vi "Build Create Parameters.vi"(4 "TypeMap in":refnum<class "TypeMap.lvclass">, 8 "error in (no error)":errorcluster, 10 "object":variant, 11 "SqlMapper in":refnum<class "SqlMapper.lvclass">) -> (0 "error out":errorcluster, 1 "DynamicParameters out":refnum<class "DynamicParameters.lvclass">, 3 "SqlMapper out":refnum<class "SqlMapper.lvclass">)   [LabVIEW 2020, in "ORM.lvlib" / "TypeMap.lvclass"]
uses:
  TypeMap.lvclass
  DynamicParameters/DynamicParameters.lvclass
  SqlMapper/SqlMapper.lvclass
  TypeMap.lvclass/TypeMap.ctl
  Read Autokey.vi
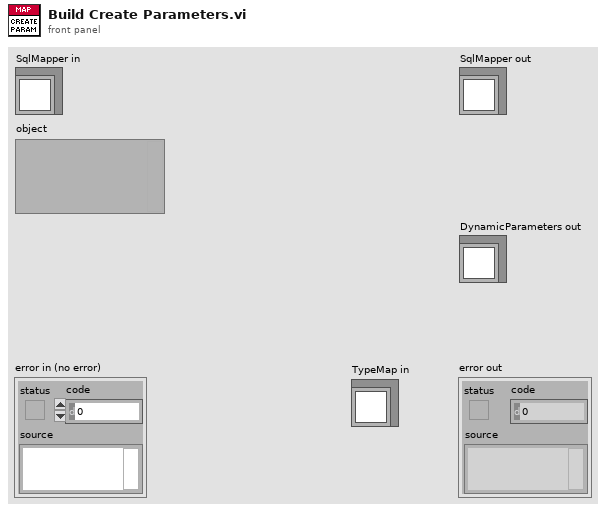
[diagram p1: front panel]
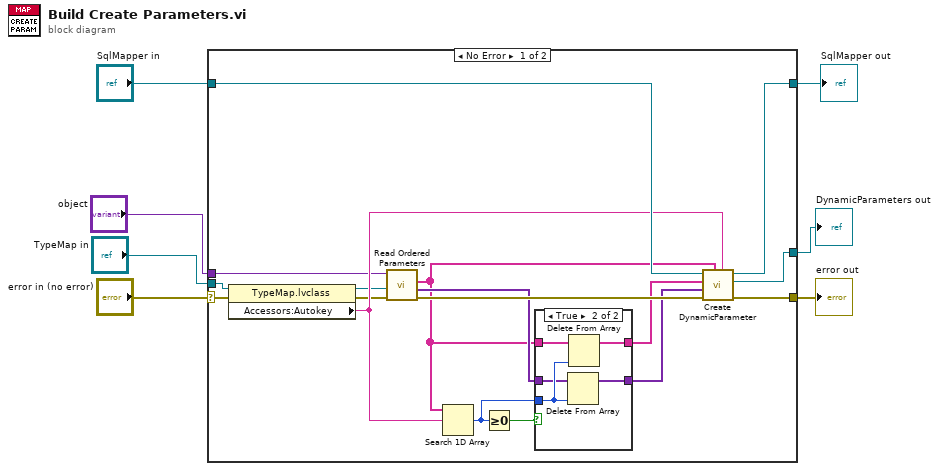
[diagram p0: block diagram]
diagram:
  n1 = case shown="No Error" "error in (no error)" {
    selector: "error in (no error)" -> [w22 w33]
    tunnel: [w14 w33] -> w6
    tunnel: "TypeMap in" -> [w24 _]
    tunnel: "object" -> [w10 _]
    tunnel: [w19 _] -> w3
    tunnel: [w20 w32] -> w2
    tunnel: "SqlMapper in" -> [w21 w32]
    frame No Error {
      n2 = property class="TypeMap.lvclass"(reference=w24, error in=w22) -> (reference out=w11:refnum<class "TypeMap.lvclass">, error out=w12:errorcluster, "Accessors:Autokey"=w13:string)
      n3 = call "Read Ordered Parameters.vi"("error in (no error)"=w12, "TypeMap in"=w11, "Object In"=w10) -> ("error out"=w23:errorcluster, "Values"=w9:variant[], "Fields"=w8:string[])  [unwired: 5 in, 1 out]
      n4 = Search 1D Array(1D array=w8, element=w13) -> (index of element=w17:i32)  [unwired: 1 in]
      n5 = Greater Or Equal To 0?(x=w17) -> (x >= 0?=w18:bool)
      n6 = case shown="True" w18 {
        tunnel: w17 -> [_ w31]
        tunnel: w8 -> [w26 w30]
        tunnel: w9 -> [w25 w29]
        tunnel: [w26 w28] -> w16
        tunnel: [w25 w27] -> w15
        frame False {
        }
        frame True {
          n7 = Delete From Array(array=w29, index=w31) -> (array with subset deleted=w27:variant[])  [unwired: 1 in, 1 out]
          n8 = Delete From Array(array=w30, index=w31) -> (array with subset deleted=w28:string[])  [unwired: 1 in, 1 out]
        }
      }
      n9 = call "Create DynamicParameter.vi"("AutoKey"=w13, "RequestedFields"=w8, "error in (no error)"=w23, "ParameterValues"=w15, "ParameterNames"=w16, "SqlMapper in"=w21) -> ("error out"=w14:errorcluster, "Parameters"=w19:refnum<class "DynamicParameters.lvclass">, "SqlMapper out"=w20:refnum<class "SqlMapper.lvclass">)  [unwired: 1 in, 2 out]
    }
    frame Error {
    }
  }
  "error out" <- w6
  "DynamicParameters out" <- w3
  "SqlMapper out" <- w2
